vi "Create Signal Properties - Sine.vi"(6 "phase":dbl format="%#_13g", 8 "error in (no error)":errorcluster, 9 "amplitude":dbl, 10 "frequency":dbl, 11 "AudioGeneration in":refnum<class "AudioGeneration.lvclass">) -> (0 "error out":errorcluster, 2 "signal settings":T1, 3 "AudioGeneration out":refnum<class "AudioGeneration.lvclass">)   [LabVIEW 2021, in "AudioGeneration.lvclass"]
uses:
  AudioGeneration.lvclass
  controls/signal settings.ctl
  controls/signal type.ctl
  controls/sine wave properties.ctl
  AudioGeneration.lvclass/AudioGeneration.ctl
  controls/AudioGenTypeDefs.lvlib
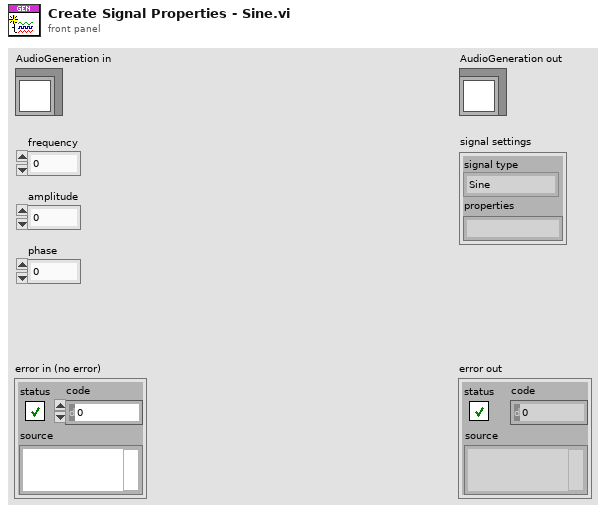
[diagram p1: front panel]
types:
  T1 = typedef "AudioGenTypeDefs.lvlib/signal settings.ctl" = cluster{"signal type":T2, "properties":string}
  T2 = typedef "AudioGenTypeDefs.lvlib/signal type.ctl" = enum16{"Sine", "Square", "Triangle", "White Noise", "Pink Noise", "Periodic Random Noise"}
  T3 = typedef "AudioGenTypeDefs.lvlib/sine wave properties.ctl" = cluster{"frequency":dbl, "amplitude":dbl, "phase":dbl}[]
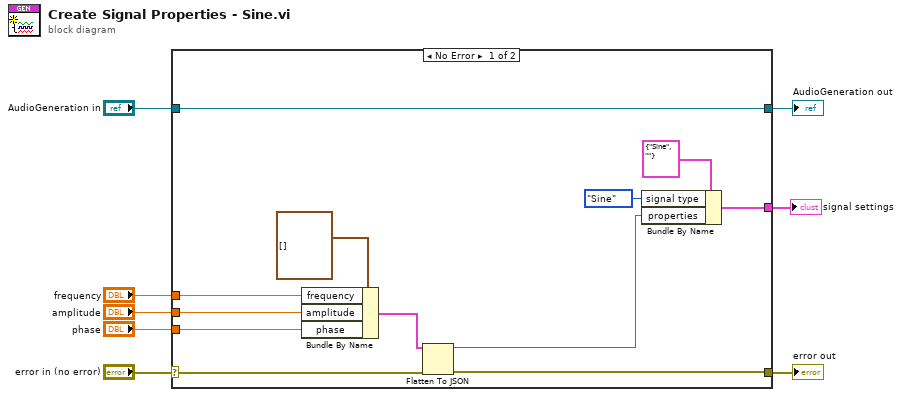
[diagram p0: block diagram]
diagram:
  n1 = case shown="No Error" "error in (no error)" {
    selector: "error in (no error)" -> [w15 w22]
    tunnel: [w12 w22] -> w7
    tunnel: [w20 w21] -> w5
    tunnel: "AudioGeneration in" -> [w20 w21]
    tunnel: [w18 _] -> w4
    tunnel: "phase" -> [w11 _]
    tunnel: "amplitude" -> [w10 _]
    tunnel: "frequency" -> [w9 _]
    frame No Error {
      n2 = Bundle By Name(cluster=T3 [] ("sine wave properties"), "frequency"=w9, "amplitude"=w10, "phase"=w11) -> (w14:cluster{})
      n3 = Flatten To JSON(anything=w14, error in (no error)=w15) -> (JSON string=w13:string, 11:w12:errorcluster)  [unwired: 1 in]
      n4 = Bundle By Name(cluster=T1 {"signal type"=enum."Sine", "properties"=""} ("signal settings"), "signal type"=signal_type."Sine", "properties"=w13) -> (w18:T1)
    }
    frame Error {
    }
  }
  "error out" <- w7
  "AudioGeneration out" <- w5
  "signal settings" <- w4
